vi "data_distributor_naive.vi"(0 "Analog Data Array In":T6[](array[typedef]), 9 "Indicies":T3[](array[typedef])=[{"Index Array"=[-1, 19, 20]}, {"Index Array"=[21]}, {"Index Array"=[5, 9, 6, 11, 7, 10, 4, 8, 4, 8, 16, -1, 14, 13, 12, 13]}, {"Index Array"=[1, 3]}, {"Index Array"=[4, 2, 0, 10, 11]}, {"Index Array"=[22, 23, 24, 29, 30, 31, 32, 25, 26, 27, 18, 17, 38, 39]}, {"Index Array"=[33, 34, 35, 31]}, {"Index Array"=[0, 1, 2, 3, 28]}], 11 "error in":errorcluster) -> (1 "Pulse Generator Charts":T5={"Vapor Mass Flow Rates"={"max value"=3.7446962566639153, "max value"=45.211135640025056}, "Test Section Thermocouples"={"[0]"=0.0, "[1]"=0.0, "[2]"=21.79653799459621, "[3]"=0.0, "[4]"=0.0}, "Pulse Generator Abs Pressure"=[132998.53122367428], "Test Section Saturation Pressures"={"max value"=57418.5, "max value"=57418.5}}, 3 "Diode Charts":T4={"Liquid Diodes"={10.35690505599997, 10.45756001099999}, "Liquid Intensity Ratio"=0.9903749101229978, "Vapor Diode"={0.0, 0.0}, "Vapor Intensity Ratio"=0.0, "TS Window 1 Temperatures"={"Average"=21.79653799459621, "T Sat [C]"=16.72998944878158}}, 6 "Measurements Data":T1={"PG Abs Pressure"=132998.53122367428, "Vapor Temperature"=21.95063222619171, "Liquid Temperature"=21.551358444754847, "PG Supply Temperature"=-40.9090848933398, "Tinlet"=21.775429293383564, "Tsectwo"=21.773893954638396, "TS Abs Pressure W1"=108233.54493510515, "TS Abs Pressure W7"=107636.14914554596, "W1-4 dP[Pa]"=15.03715457001021, "W1-7 dP[Pa]"=-11.039432861497964, "W1-7 dP[Pa] Fast"=6.305384010424721, "PG Venturi dP [Pa]"=13.253988595884472, "Vapor Line Pitot dP [Pa]"=1890.5846161976224, "Tsecthree"=21.74813177970565, "Toutlet"=21.728485158190438, "TS Ext"=18.97439824494449, "Vapor Sat Pressure"=131468.6007873703, "Liquid Sat Pressure"=129502.44131353268, "PG Mass Flow Rate"=3.7446962566639153, "Vapor Line Mass Flow"=45.211135640025056}, 10 "Pressure/Temperature/Mixture Properties":T2={"Line Densities\n[g/cm^3]"={"Vapor Line"=1.344129471, "Liquid Line"=1.34048179555625}, "Mixture Properties"={"Enthalpy"=301805.12673291145, "Quality [-]"=0.3812094806949553}, "Component PTs"={"Liquid Tank P"=167112.5779744949, "Liquid Tank T"=21.84509799786669, "Liquid Tank Sat P"=130946.03056847634, "Liquid Tank Sat T"=28.610704130478283, "Separator P"=132369.9601656734, "Separator T"=22.078885751559927, "Separator Sat P"=132106.4773606729, "Separator Sat T"=22.236042708091574, "Liquid Inlet P"=119629.0690348441, "Liquid Inlet T"=22.085674347190754, "Liquid Inlet Sat P"=132140.32695954802, "Liquid Inlet Sat T"=19.46796815858083, "Vapor Tank P"=87375.53249129167, "Vapor Tank T"=22.56105126295147, "Vapor Tank Sat P"=134532.36915875768, "Vapor Tank Sat T"=10.87475257267468, "Vapor Inlet P"=87375.53249129167, "Vapor Inlet T"=22.56105126295147, "Vapor Inlet Sat P"=134532.36915875768, "Vapor Inlet Sat T"=10.87475257267468, "Test Section P"=98782.87454816521, "Test Section T"=0.0, "Test Section Sat P"=57418.5, "Test Section Sat T"=14.23098988874186, "Upper Dev Section P"=109868.41958658777, "Upper Dev Section T"=21.62616176270025, "Upper Dev Section Sat P"=129868.54644319683, "Upper Dev Section Sat T"=17.14004188643561, "Lower Dev Section P"=120439.80500464814, "Lower Dev Section T"=21.62616176270025, "Lower Dev Section Sat P"=129868.54644319683, "Lower Dev Section Sat T"=19.65270419356638}, "Ambient Pressure [Pa]"=97587.26923397348, "Mixing Tee"={"Venturi dP"=0.0, "PGminiPressure"=97328.4990998598, "PGminiTemperature"=22.452186094046652}}, 12 "Vapor Flow":cluster{"Average":dbl, "Average":dbl}={"Average"=-0.36685070943632087, "Average"=1.344129471}, 13 "Liquid Flow":cluster{"Average":dbl, "Average":dbl}={"Average"=-0.6100773897297921, "Average"=1.34048179555625}, 14 "CameraVoltage":dbl[](array[numeric])=[10.439056993, 10.439056993, 10.439056993, 10.439056993, 10.439056993, 10.439056993, 10.439056993, 10.439056993, 10.439056993, 10.439056993, 10.439056993, 10.439056993, 10.439056993, 10.439056993, 10.439056993, 10.439056993, 10.439056993, 10.439056993, 10.439056993, 10.439056993, 10.439056993, 10.439056993, 10.439056993, 10.439056993, 10.439056993, 10.439056993, 10.439056993, 10.439056993, 10.439056993, 10.439056993, 10.439056993, 10.439056993, 10.439056993, 10.439056993, 10.439056993, 10.439056993, 10.439056993, 10.439056993, 10.439056993, 10.439056993, 10.439056993, 10.439056993, 10.439056993, 10.439056993, 10.439056993, 10.439056993, 10.439056993, 10.439056993, 10.439056993, 10.439056993, 10.439056993, 10.439056993, 10.439056993, 10.439056993, 10.439056993, 10.439056993, 10.439056993, 10.439056993, 10.439056993, 10.439056993, 10.439056993, 10.439056993, 10.439056993, 10.439056993, 10.439056993, 10.439056993, 10.439056993, 10.439056993, 10.439056993, 10.439056993, 10.439056993, 10.439056993, 10.439056993, 10.439056993, 10.439056993, 10.439056993, 10.439056993, 10.439056993, 10.439056993, 10.439056993, 10.439056993, 10.439056993, 10.439056993, 10.439056993, 10.439056993, 10.439056993, 10.439056993, 10.439056993, 10.439056993, 10.439056993, 10.439056993, 10.439056993, 10.439056993, 10.439056993, 10.439056993, 10.439056993, 10.439056993, 10.439056993, 10.439056993, 10.439056993, 10.439056993, 10.439056993, 10.439056993, 10.439056993, 10.439056993, 10.439056993, 10.439056993, 10.439056993, 10.439056993, 10.439056993, 10.439056993, 10.439056993, 10.439056993, 10.439056993, 10.439056993, 10.439056993, 10.439056993, 10.439056993, 10.439056993, 10.439056993, 10.439056993, 10.439056993, 10.439056993, 10.439056993, 10.439056993, 10.439056993, 10.439056993, 10.439056993, 10.439056993, 10.439056993, 10.439056993, 10.439056993, 10.439056993, 10.439056993, 10.439056993, 10.439056993, 10.439056993, 10.439056993, 10.439056993, 10.439056993, 10.439056993, 10.439056993, 10.439056993, 10.439056993, 10.439056993, 10.439056993, 10.439056993, 10.439056993, 10.439056993, 10.439056993, 10.439056993, 10.439056993, 10.439056993, 10.439056993, 10.439056993, 10.439056993, 10.439056993, 10.439056993, 10.439056993, 10.439056993, 10.439056993, 10.439056993, 10.439056993, 10.439056993, 10.439056993, 10.439056993, 10.439056993, 10.439056993, 10.439056993, 10.439056993, 10.439056993, 10.439056993, 10.439056993, 10.439056993, 10.439056993, 10.439056993, 10.439056993, 10.439056993, 10.439056993, 10.439056993, 10.439056993, 10.439056993, 10.439056993, 10.439056993, 10.439056993, 10.439056993, 10.439056993, 10.439056993, 10.439056993, 10.439056993, 10.439056993, 10.439056993, 10.439056993, 10.439056993, 10.439056993, 10.439056993, 10.439056993, 10.439056993, 10.439056993, 10.439056993], 15 "error out":errorcluster)   [LabVIEW 2022 SP3]
uses:
  analog_data.ctl
  Utility Sub VIs/pulse_generator_data_charts.ctl
  Utility Sub VIs/diode_charts.ctl
  index_array_cluster.ctl
  Utility Sub VIs/pressure_temp_mixture.ctl
  Utility Sub VIs/pulse_generator_data.ctl
panel:
  # "Test Section"
  # "Pulse Gen"
  # "Saturation\nPressure [Pa]"
  # "Saturation\nTemperature [C]"
  # "Pressure [Pa]"
  # "Temperature [C]"
  # "Liquid Tank"
  # "Separator"
  # "Liquid Inlet"
  # "Vapor Tank"
  # "Vapor Inlet"
  # "Test Section"
  # "Upper Dev Section"
  # "Lower Dev Section"
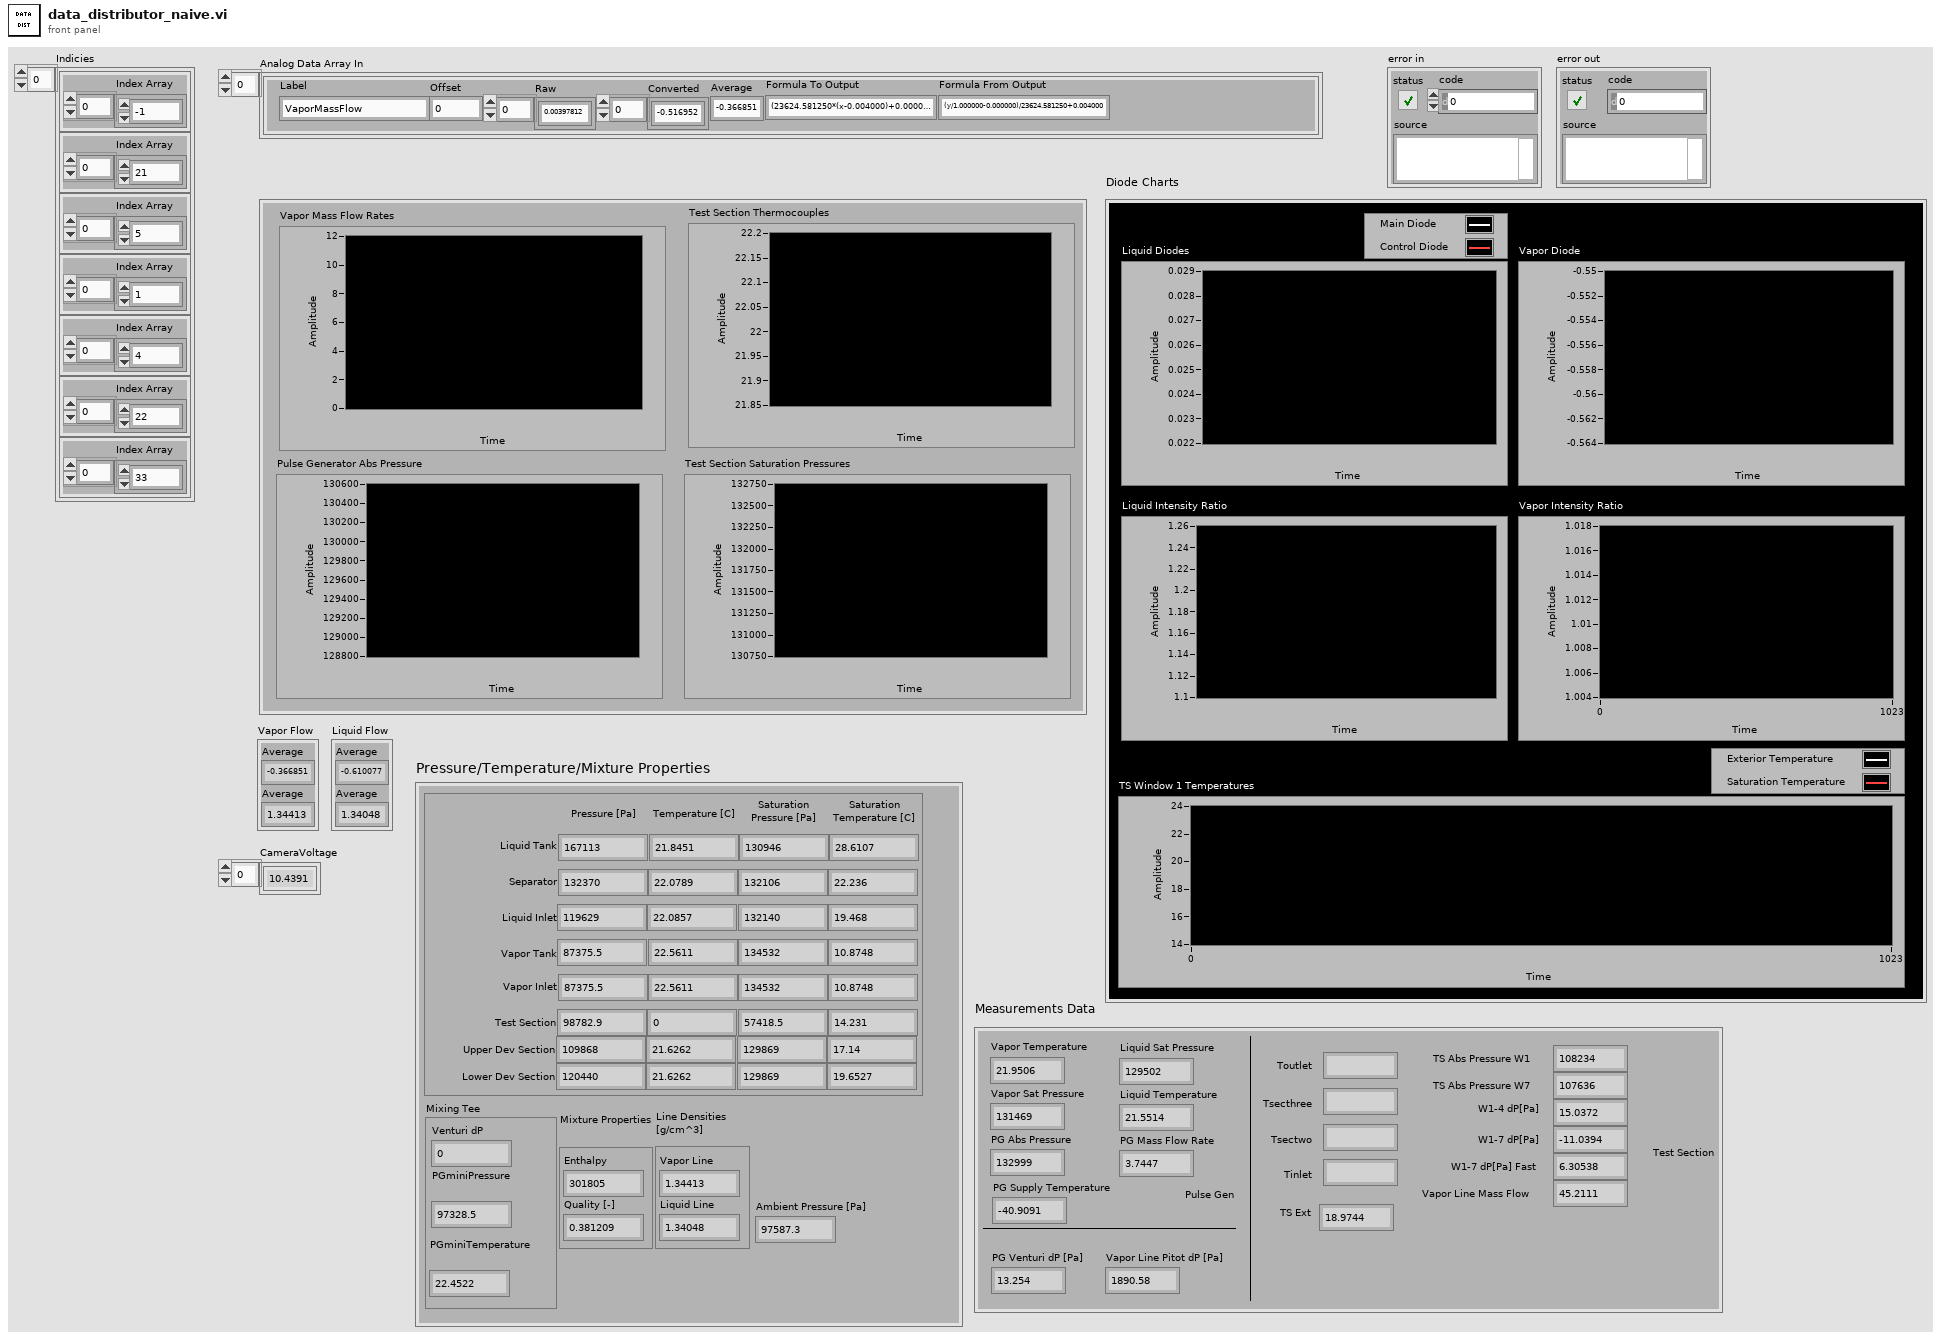
[diagram p1: front panel]
types:
  T1 = typedef "pulse_generator_data.ctl" = cluster{"PG Abs Pressure":dbl, "Vapor Temperature":dbl, "Liquid Temperature":dbl, "PG Supply Temperature":dbl, "Tinlet":dbl, "Tsectwo":dbl, "TS Abs Pressure W1":dbl, "TS Abs Pressure W7":dbl, "W1-4 dP[Pa]":dbl, "W1-7 dP[Pa]":dbl, "W1-7 dP[Pa] Fast":dbl, "PG Venturi dP [Pa]":dbl, "Vapor Line Pitot dP [Pa]":dbl, "Tsecthree":dbl, "Toutlet":dbl, "TS Ext":dbl, "Vapor Sat Pressure":dbl, "Liquid Sat Pressure":dbl, "PG Mass Flow Rate":dbl, "Vapor Line Mass Flow":dbl}
  T2 = typedef "pressure_temp_mixture.ctl" = cluster{"Line Densities\n[g/cm^3]":cluster{"Vapor Line":dbl, "Liquid Line":dbl}, "Mixture Properties":cluster{"Enthalpy":dbl, "Quality [-]":dbl}, "Component PTs":cluster{"Liquid Tank P":dbl, "Liquid Tank T":dbl, "Liquid Tank Sat P":dbl, "Liquid Tank Sat T":dbl, "Separator P":dbl, "Separator T":dbl, "Separator Sat P":dbl, "Separator Sat T":dbl, "Liquid Inlet P":dbl, "Liquid Inlet T":dbl, "Liquid Inlet Sat P":dbl, "Liquid Inlet Sat T":dbl, "Vapor Tank P":dbl, "Vapor Tank T":dbl, "Vapor Tank Sat P":dbl, "Vapor Tank Sat T":dbl, "Vapor Inlet P":dbl, "Vapor Inlet T":dbl, "Vapor Inlet Sat P":dbl, "Vapor Inlet Sat T":dbl, "Test Section P":dbl, "Test Section T":dbl, "Test Section Sat P":dbl, "Test Section Sat T":dbl, "Upper Dev Section P":dbl, "Upper Dev Section T":dbl, "Upper Dev Section Sat P":dbl, "Upper Dev Section Sat T":dbl, "Lower Dev Section P":dbl, "Lower Dev Section T":dbl, "Lower Dev Section Sat P":dbl, "Lower Dev Section Sat T":dbl}, "Ambient Pressure [Pa]":dbl, "Mixing Tee":cluster{"Venturi dP":dbl, "PGminiPressure":dbl, "PGminiTemperature":dbl}}
  T3 = typedef "index_array_cluster.ctl" = cluster{"Index Array":i32[]}
  T4 = typedef "diode_charts.ctl" = cluster{"Liquid Diodes":cluster{dbl, dbl}, "Liquid Intensity Ratio":dbl, "Vapor Diode":cluster{dbl, dbl}, "Vapor Intensity Ratio":dbl, "TS Window 1 Temperatures":cluster{"Average":dbl, "T Sat [C]":dbl}}
  T5 = typedef "pulse_generator_data_charts.ctl" = cluster{"Vapor Mass Flow Rates":cluster{"max value":dbl, "max value":dbl}, "Test Section Thermocouples":cluster{"[0]":dbl, "[1]":dbl, "[2]":dbl, "[3]":dbl, "[4]":dbl}, "Pulse Generator Abs Pressure":dbl[], "Test Section Saturation Pressures":cluster{"max value":dbl, "max value":dbl}}
  T6 = typedef "analog_data.ctl" = cluster{"Label":string, "Offset":dbl, "Raw":dbl[], "Converted":dbl[], "Average":dbl, "Formula To Output":string, "Formula From Output":string}
  T7 = cluster{"Mixing Tee dP":dbl, "PG inlet-Mixing Tee Abs Pressure":dbl, "PG inlet-Mixing Tee Temperature":dbl}
  T8 = cluster{"[0]":dbl, "[1]":dbl, "[2]":dbl, "[3]":dbl, "[4]":dbl, "[5]":dbl, "[6]":dbl, "[7]":dbl, "[8]":dbl, "[9]":dbl, "[10]":dbl, "[11]":dbl, "[12]":dbl, "[13]":dbl, "[14]":dbl, "[15]":dbl, "[16]":dbl, "[17]":dbl, "[18]":dbl, "[19]":dbl, "[20]":dbl, "[21]":dbl, "[22]":dbl, "[23]":dbl, "[24]":dbl, "[25]":dbl, "[26]":dbl, "[27]":dbl, "[28]":dbl, "[29]":dbl, "[30]":dbl, "[31]":dbl}
  T9 = cluster{"Mass Flow Rate [g/s]":dbl, "Mass Flow Rate [g/s]":dbl}
  T10 = cluster{"[0]":dbl, "[1]":dbl, "[2]":dbl, "[3]":dbl, "[4]":dbl}
  T11 = cluster{"[0]":dbl, "[1]":dbl, "[2]":dbl, "[3]":dbl, "[4]":dbl, "[5]":dbl, "[6]":dbl, "[7]":dbl, "[8]":dbl, "[9]":dbl, "[10]":dbl, "[11]":dbl, "[12]":dbl, "[13]":dbl, "[14]":dbl, "[15]":dbl, "[16]":dbl, "[17]":dbl, "[18]":dbl, "[19]":dbl}
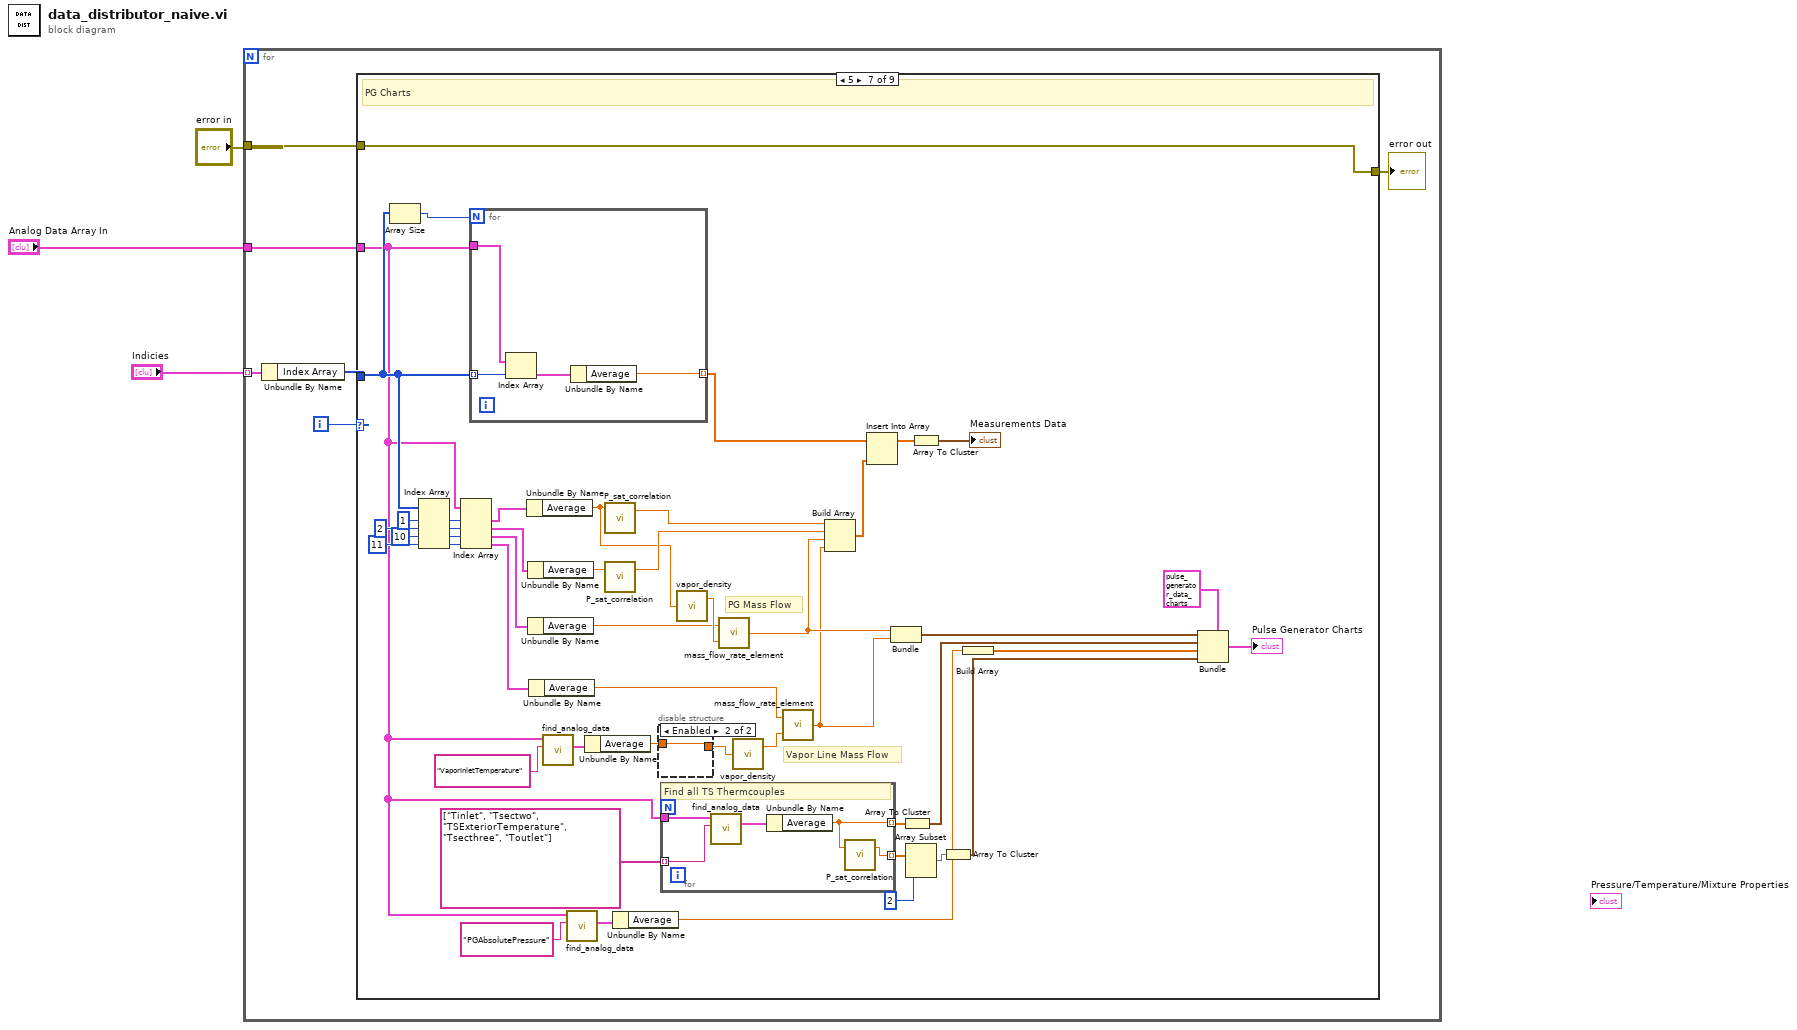
[diagram p0: block diagram]
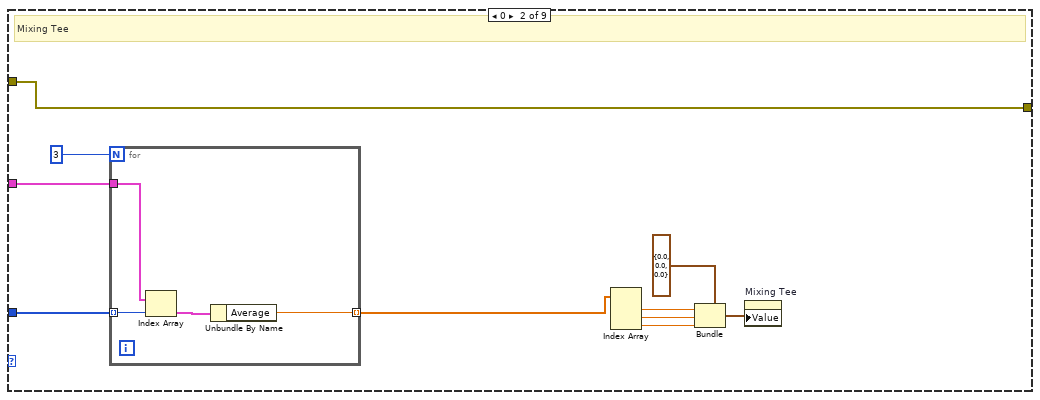
[diagram p3: hidden frame]
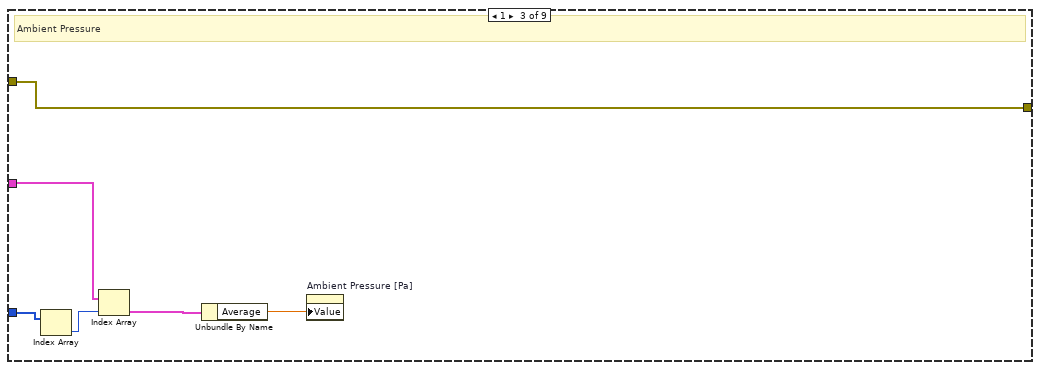
[diagram p4: hidden frame]
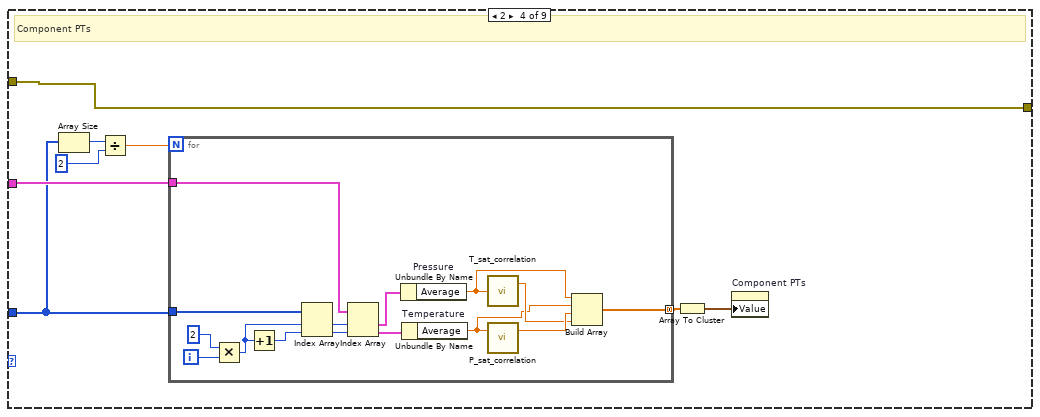
[diagram p5: hidden frame]
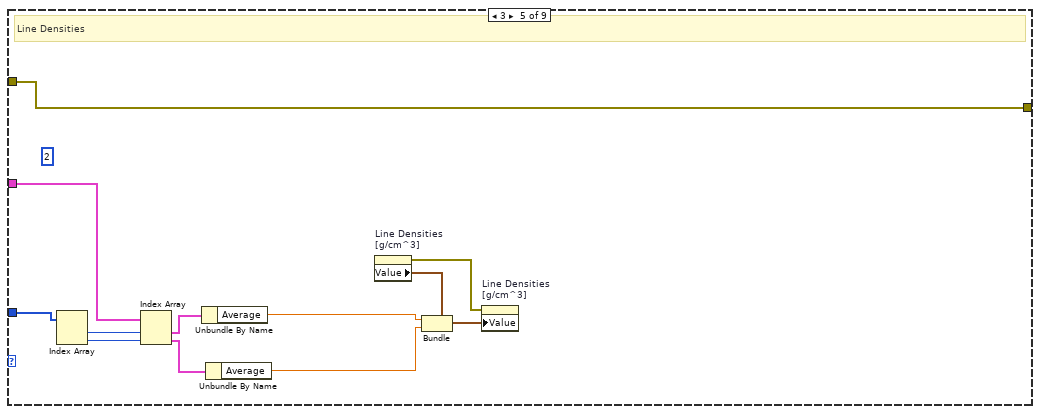
[diagram p6: hidden frame]
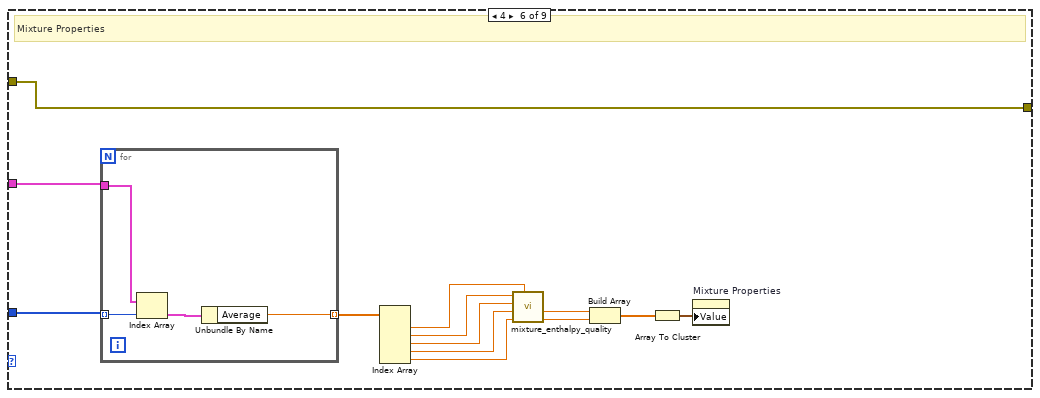
[diagram p7: hidden frame]
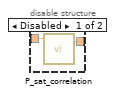
[diagram p8: hidden frame]
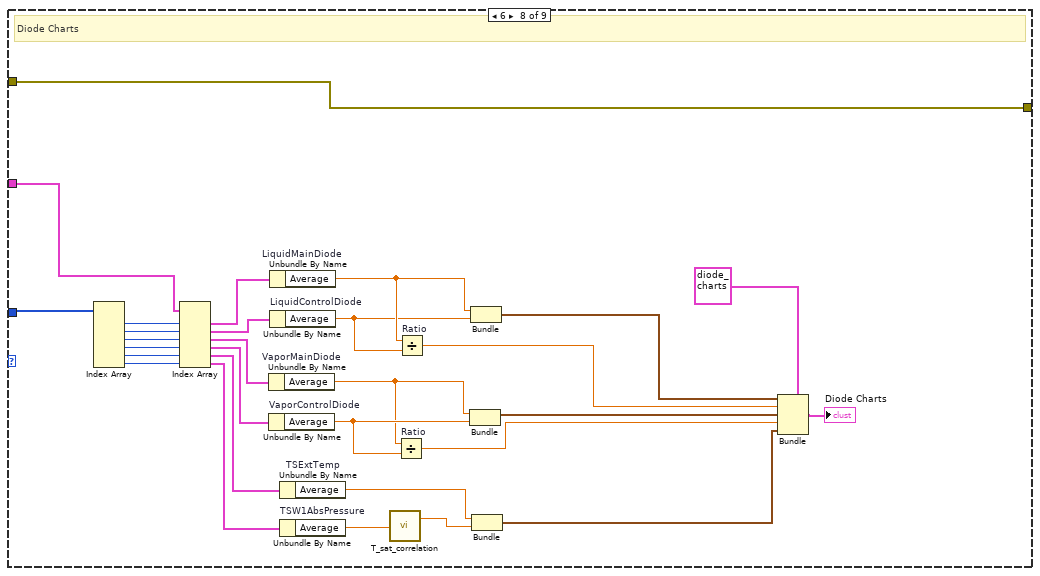
[diagram p9: hidden frame]
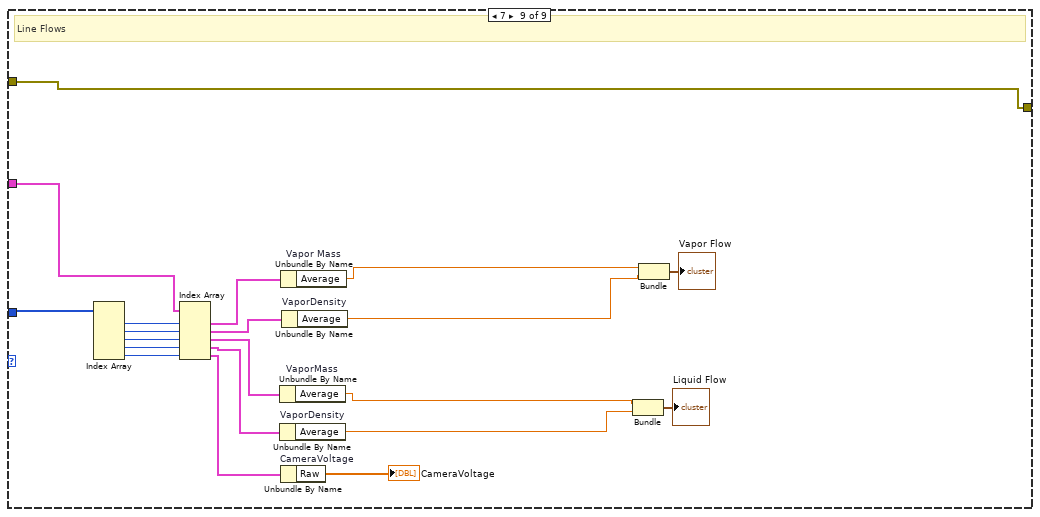
[diagram p10: hidden frame]
diagram:
  n1 = for {
    tunnel: "error in" -> [w9]
    tunnel: "Analog Data Array In" -> [w8]
    tunnel: "Indicies" -> [w5] mode=indexing
    i -> [w4]
    n2 = Unbundle By Name(w5) -> ("Index Array"=w6:i32[])
    n3 = case shown="5" w4 {
      tunnel: w6 -> [_ w20 w28 w37 w62 w77 w102 w171 w191]
      tunnel: w8 -> [_ w19 w30 w38 w59 w78 w92 w169 w189]
      tunnel: w9 -> [w10 w12 w26 w32 w63 w67 w103 w158 w177]
      tunnel: [w10 w12 w26 w32 w63 w67 w103 w158 w177] -> w7
      frame Default {
      }
      frame 0 {
        # "Mixing Tee"
        n4 = for {
          N: 3 -> [_]
          tunnel: w20 -> [w24] mode=indexing
          tunnel: w19 -> [w23]
          tunnel: [w21] -> w17 mode=indexing
          n5 = Index Array(array=w23, index=w24) -> (element=w22:T6)
          n6 = Unbundle By Name(w22) -> ("Average"=w21:dbl)
        }
        n7 = Index Array(array=w17) -> (element #1=w15:dbl, element #2=w14:dbl, element #3=w13:dbl)  [unwired: 3 in]
        n8 = Bundle(cluster=T7 {"Mixing Tee dP"=0.0, "PG inlet-Mixing Tee Abs Pressure"=0.0, "PG inlet-Mixing Tee Temperature"=0.0} ("Mixing Tee"), "Mixing Tee dP"=w15, "PG inlet-Mixing Tee Abs Pressure"=w14, "PG inlet-Mixing Tee Temperature"=w13) -> (w11:T7)
        n9 = property on="Mixing Tee" class="Clust (strict)"("Value"=w11) -> ()  [unwired: 2 in, 2 out]
      }
      frame 1 {
        # "Ambient Pressure"
        n10 = Index Array(array=w28) -> (element=w27:i32)  [unwired: 1 in]
        n11 = Index Array(array=w30, index=w27) -> (element=w29:T6)
        n12 = Unbundle By Name(w29) -> ("Average"=w25:dbl)
        n13 = property on="Ambient Pressure [Pa]" class="DigNum (strict)"("Value"=w25) -> ()  [unwired: 2 in, 2 out]
      }
      frame 2 {
        # "Component PTs"
        n14 = Array Size(array=w37) -> (size(s)=w35:i32)
        n15 = Divide(x=w35, y=2) -> (x/y=w36:dbl)
        n16 = for {
          N: w36 -> [_]
          tunnel: w37 -> [w49]
          tunnel: w38 -> [w53]
          tunnel: [w39] -> w33 mode=concatenating
          i -> [w51]
          n17 = Multiply(x=2, y=w51) -> (x*y=w47:i32)
          n18 = Increment(x=w47) -> (x+1=w48:i32)
          n19 = Index Array(array=w49, index #1=w47, index #2=w48) -> (element #1=w46:i32, element #2=w45:i32)
          n20 = Index Array(array=w53, index #1=w46, index #2=w45) -> (element #1=w52:T6, element #2=w44:T6)
          n21 = Unbundle By Name "Pressure"(w52) -> ("Average"=w41:dbl)
          n22 = Unbundle By Name "Temperature"(w44) -> ("Average"=w40:dbl)
          n23 = call "T_sat_correlation.vi"("P [Pa]"=w41) -> ("T Sat [C]"=w42:dbl)  [unwired: 1 out]
          n24 = call "P_sat_correlation.vi"("Temperature[C]"=w40) -> ("P Sat[Pa]"=w43:dbl)  [unwired: 1 in, 1 out]
          n25 = Build Array(w41, w40, w43, w42) -> (w39:dbl[])
        }
        n26 = Array To Cluster(array=w33) -> (cluster=w31:T8)
        n27 = property on="Component PTs" class="Clust (strict)"("Value"=w31) -> ()  [unwired: 2 in, 2 out]
      }
      frame 3 {
        (unwired) 2
        # "Line Densities"
        n28 = Index Array(array=w62) -> (element #1=w60:i32, element #2=w61:i32)  [unwired: 2 in]
        n29 = Index Array(array=w59, index #1=w60, index #2=w61) -> (element #1=w58:T6, element #2=w57:T6)
        n30 = Unbundle By Name(w58) -> ("Average"=w65:dbl)
        n31 = Unbundle By Name(w57) -> ("Average"=w64:dbl)
        n32 = property on="Line Densities\n[g/cm^3]" class="Clust (strict)"() -> (error out=w55:errorcluster, "Value"=w54:cluster{"Vapor Line":dbl, "Liquid Line":dbl})  [unwired: 2 in, 1 out]
        n33 = Bundle(cluster=w54, "Vapor Line"=w65, "Liquid Line"=w64) -> (w56:cluster{"Vapor Line":dbl, "Liquid Line":dbl})
        n34 = property on="Line Densities\n[g/cm^3]" class="Clust (strict)"(error in=w55, "Value"=w56) -> ()  [unwired: 1 in, 2 out]
      }
      frame 4 {
        # "Mixture Properties"
        n35 = for {
          tunnel: w77 -> [w82] mode=indexing
          tunnel: w78 -> [w81]
          tunnel: [w79] -> w76 mode=indexing
          n36 = Index Array(array=w81, index=w82) -> (element=w80:T6)
          n37 = Unbundle By Name(w80) -> ("Average"=w79:dbl)
        }
        n38 = Index Array(array=w76) -> (element #1=w72:dbl, element #2=w71:dbl, element #3=w70:dbl, element #4=w69:dbl, element #5=w68:dbl)  [unwired: 5 in]
        n39 = call "mixture_enthalpy_quality.vi"("Vapor Inlet Pressure [Pa]"=w72, "Separator Temp [C]"=w68, "Liquid Inlet Temp [C]"=w69, "Vapor Flow Rate [g/s]"=w70, "Liquid Flow Rate [g/s]"=w71) -> ("Quality [-]"=w74:dbl, "mixture enthalpy"=w75:dbl)  [unwired: 2 out]
        n40 = Build Array(w75, w74) -> (w73:dbl[])
        n41 = Array To Cluster(array=w73) -> (cluster=w66:cluster{"[0]":dbl, "[1]":dbl})
        n42 = property on="Mixture Properties" class="Clust (strict)"("Value"=w66) -> ()  [unwired: 2 in, 2 out]
      }
      frame 5 {
        # "Vapor Line Mass Flow"
        # "PG Mass Flow"
        # "PG Charts"
        n43 = Array Size(array=w102) -> (size(s)=w109:i32)
        n44 = Index Array(array=w102, index #1=1 ("index"), index #2=2 ("index"), index #3=10 ("index"), index #4=11 ("index")) -> (element #1=w101:i32, element #2=w96:i32, element #3=w95:i32, element #4=w94:i32)
        n45 = Index Array(array=w92, index #1=w101, index #2=w96, index #3=w95, index #4=w94) -> (element #1=w93:T6, element #2=w91:T6, element #3=w90:T6, element #4=w89:T6)
        n46 = for {
          N: w109 -> [_]
          tunnel: w102 -> [w142] mode=indexing
          tunnel: w92 -> [w141]
          tunnel: [w139] -> w122 mode=indexing
          n47 = Index Array(array=w141, index=w142) -> (element=w140:T6)
          n48 = Unbundle By Name(w140) -> ("Average"=w139:dbl)
        }
        n49 = Unbundle By Name(w93) -> ("Average"=w110:dbl)
        n50 = Unbundle By Name(w91) -> ("Average"=w130:dbl)
        n51 = Unbundle By Name(w90) -> ("Average"=w83:dbl)
        n52 = Unbundle By Name(w89) -> ("Average"=w123:dbl)
        n53 = call "find_analog_data.vi"("Needle"="VaporInletTemperature", "Haystack"=w92) -> ("Needle Out"=w127:T6)  [unwired: 7 in, 2 out]
        n54 = call "find_analog_data.vi"("Needle"="PGAbsolutePressure", "Haystack"=w92) -> ("Needle Out"=w116:T6)  [unwired: 7 in, 2 out]
        n55 = Unbundle By Name(w127) -> ("Average"=w126:dbl)
        n56 = call "P_sat_correlation.vi"("Temperature[C]"=w110) -> ("P Sat[Pa]"=w121:dbl)  [unwired: 1 in, 1 out]
        n57 = call "P_sat_correlation.vi"("Temperature[C]"=w130) -> ("P Sat[Pa]"=w120:dbl)  [unwired: 1 in, 1 out]
        n58 = Unbundle By Name(w116) -> ("Average"=w115:dbl)
        n59 = disable-structure shown="Enabled" {
          disable-tunnel: w126 -> [w132 w133]
          disable-tunnel: [w131 w133] -> w125
          frame Disabled {
            n60 = call "P_sat_correlation.vi"("Temperature[C]"=w132) -> ("P Sat[Pa]"=w131:dbl)  [unwired: 1 in, 1 out]
          }
          frame Enabled {
          }
        }
        n61 = for {
          tunnel: string[] ["Tinlet", "Tsectwo", "TSExteriorTemperature", "Tsecthree", "Toutlet"] ("Needle") -> [w137] mode=indexing
          tunnel: w92 -> [w138]
          tunnel: [w135] -> w111 mode=indexing
          tunnel: [w134] -> w87 mode=indexing
          # "Find all TS Thermcouples"
          n62 = call "find_analog_data.vi"("Needle"=w137, "Haystack"=w138) -> ("Needle Out"=w136:T6)  [unwired: 7 in, 2 out]
          n63 = Unbundle By Name(w136) -> ("Average"=w135:dbl)
          n64 = call "P_sat_correlation.vi"("Temperature[C]"=w135) -> ("P Sat[Pa]"=w134:dbl)  [unwired: 1 in, 1 out]
        }
        n65 = call "vapor_density.vi"("Vapor Temp [C]"=w110) -> ("Vapor Density[g/cm3]"=w129:dbl)  [unwired: 1 out]
        n66 = call "mass_flow_rate_element.vi"("Density [g/cm3]"=w129, "dP [Pa]"=w83) -> ("Mass Flow Rate [g/s]"=w114:dbl)
        n67 = call "vapor_density.vi"("Vapor Temp [C]"=w125) -> ("Vapor Density[g/cm3]"=w124:dbl)  [unwired: 1 out]
        n68 = call "mass_flow_rate_element.vi"("Density [g/cm3]"=w124, "dP [Pa]"=w123) -> ("Mass Flow Rate [g/s]"=w113:dbl)
        n69 = Build Array(w121, w120, w114, w113) -> (w119:dbl[])
        n70 = Insert Into Array(array=w122, new element=w119) -> (w118:dbl[])  [unwired: 1 in]
        n71 = Bundle("Mass Flow Rate [g/s]"=w114, "Mass Flow Rate [g/s]"=w113) -> (w106:T9)  [unwired: 1 in]
        n72 = Array To Cluster(array=w111) -> (cluster=w84:T10)
        n73 = Array Subset(array=w87, length=2) -> (w85:dbl[])  [unwired: 1 in]
        n74 = Array To Cluster(array=w118) -> (cluster=→"Measurements Data":T11)
        n75 = Array To Cluster(array=w85) -> (cluster=w104:cluster{"[0]":dbl, "[1]":dbl})
        n76 = Build Array(w115) -> (w105:dbl[])
        n77 = Bundle(cluster=T5 {"Vapor Mass Flow Rates"={"max value"=119484.80284900061, "max value"=11360.460004869077}, "Test Section Thermocouples"={"[0]"=0.0, "[1]"=0.0, "[2]"=0.0, "[3]"=0.0, "[4]"=0.0}, "Pulse Generator Abs Pressure"=[], "Test Section Saturation Pressures"={"max value"=0.0, "max value"=0.0}} ("Pulse Generator Charts 2"), "Vapor Mass Flow Rates"=w106, "Test Section Thermocouples"=w84, "Pulse Generator Abs Pressure"=w105, "Test Section Saturation Pressures"=w104) -> (→"Pulse Generator Charts":T5)
      }
      frame 6 {
        # "Diode Charts"
        n78 = Index Array(array=w171) -> (element #1=w166:i32, element #2=w170:i32, element #3=w168:i32, element #4=w167:i32, element #5=w153:i32, element #6=w152:i32)  [unwired: 6 in]
        n79 = Index Array(array=w169, index #1=w166, index #2=w170, index #3=w168, index #4=w167, index #5=w153, index #6=w152) -> (element #1=w165:T6, element #2=w164:T6, element #3=w149:T6, element #4=w148:T6, element #5=w154:T6, element #6=w155:T6)
        n80 = Unbundle By Name "VaporMainDiode"(w149) -> ("Average"=w150:dbl)
        n81 = Unbundle By Name "VaporControlDiode"(w148) -> ("Average"=w151:dbl)
        n82 = Unbundle By Name "LiquidMainDiode"(w165) -> ("Average"=w163:dbl)
        n83 = Unbundle By Name "LiquidControlDiode"(w164) -> ("Average"=w162:dbl)
        n84 = Unbundle By Name "TSExtTemp"(w154) -> ("Average"=w160:dbl)
        n85 = Unbundle By Name "TSW1AbsPressure"(w155) -> ("Average"=w161:dbl)
        n86 = call "T_sat_correlation.vi"("P [Pa]"=w161) -> ("T Sat [C]"=w159:dbl)  [unwired: 1 out]
        n87 = Divide "Ratio"(x=w150, y=w151) -> (x/y=w145:dbl)
        n88 = Divide "Ratio"(x=w163, y=w162) -> (x/y=w156:dbl)
        n89 = Bundle("Average"=w150, "Average"=w151) -> (w146:cluster{"Average":dbl, "Average":dbl})  [unwired: 1 in]
        n90 = Bundle("Average"=w163, "Average"=w162) -> (w157:cluster{"Average":dbl, "Average":dbl})  [unwired: 1 in]
        n91 = Bundle("Average"=w160, "T Sat [C]"=w159) -> (w147:cluster{"Average":dbl, "T Sat [C]":dbl})  [unwired: 1 in]
        n92 = Bundle(cluster=T4 {"Liquid Diodes"={0.0, 0.0}, "Liquid Intensity Ratio"=0.0, "Vapor Diode"={0.0, 0.0}, "Vapor Intensity Ratio"=0.0, "TS Window 1 Temperatures"={"Average"=0.0, "T Sat [C]"=0.0}} ("Diode Charts"), "Liquid Diodes"=w157, "Liquid Intensity Ratio"=w156, "Vapor Diode"=w146, "Vapor Intensity Ratio"=w145, "TS Window 1 Temperatures"=w147) -> (→"Diode Charts":T4)
      }
      frame 7 {
        # "Line Flows"
        n93 = Index Array(array=w191) -> (element #1=w186:i32, element #2=w190:i32, element #3=w188:i32, element #4=w187:i32, element #5=w172:i32)  [unwired: 5 in]
        n94 = Index Array(array=w189, index #1=w186, index #2=w190, index #3=w188, index #4=w187, index #5=w172) -> (element #1=w185:T6, element #2=w184:T6, element #3=w183:T6, element #4=w182:T6, element #5=w174:T6)
        n95 = Unbundle By Name "VaporMass"(w183) -> ("Average"=w179:dbl)
        n96 = Unbundle By Name "VaporDensity"(w182) -> ("Average"=w178:dbl)
        n97 = Unbundle By Name "Vapor Mass"(w185) -> ("Average"=w181:dbl)
        n98 = Unbundle By Name "CameraVoltage"(w174) -> ("Raw"=→"CameraVoltage":dbl[])
        n99 = Unbundle By Name "VaporDensity"(w184) -> ("Average"=w180:dbl)
        n100 = Bundle("Average"=w179, "Average"=w178) -> (→"Liquid Flow":cluster{"Average":dbl, "Average":dbl})  [unwired: 1 in]
        n101 = Bundle("Average"=w181, "Average"=w180) -> (→"Vapor Flow":cluster{"Average":dbl, "Average":dbl})  [unwired: 1 in]
      }
    }
    "error out" <- w7
  }
